vi "Get Control Absolute Position.vi"(8 "error in (no error)":errorcluster, 11 "Boolean in":refnum<vi>) -> (0 "error out":errorcluster, 2 "Absolute Position":T1)   [LabVIEW 2017, in "Hamburger Menu Library.lvlib"]
uses:
  Hamburger Menu Library.lvlib
  <vilib>/Utility/miscctls.llb/LVPositionTypeDef.ctl
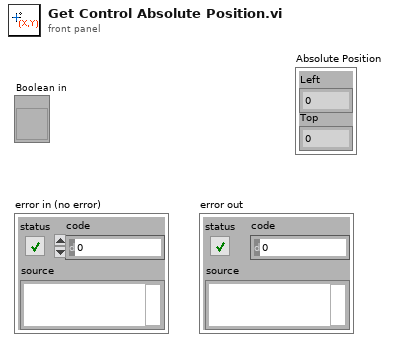
[diagram p1: front panel]
types:
  T1 = typedef "LVPositionTypeDef.ctl" = cluster{"Left":i32, "Top":i32}
  T2 = typedef "LVPointTypeDef.ctl" = cluster{"Horizontal":i16, "Vertical":i16}
  T3 = typedef "LVRectTypeDef.ctl" = cluster{"Left":i16, "Top":i16, "Right":i16, "Bottom":i16}
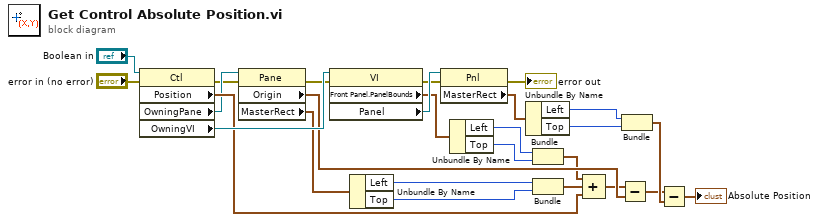
[diagram p0: block diagram]
diagram:
  n1 = property class="Ctl"(reference="Boolean in", error in="error in (no error)") -> (error out=w3:errorcluster, "Position"=w11:T1, "OwningPane"=w6:refnum<vi>, "OwningVI"=w22:refnum<vi>)  [unwired: 1 out]
  n2 = property class="Pane"(reference=w6, error in=w3) -> (error out=w2:errorcluster, "Origin"=w17:T2, "MasterRect"=w12:T3)  [unwired: 1 out]
  n3 = property class="VI"(reference=w22, error in=w2) -> (error out=w1:errorcluster, "Front Panel.PanelBounds"=w5:T3, "Panel"=w23:refnum<vi>)  [unwired: 1 out]
  n4 = Unbundle By Name(w12) -> ("Left"=w13:i16, "Top"=w14:i16)
  n5 = property class="Pnl"(reference=w23, error in=w1) -> (error out=→"error out":errorcluster, "MasterRect"=w21:T3)  [unwired: 1 out]
  n6 = Unbundle By Name(w5) -> ("Left"=w7:i16, "Top"=w8:i16)
  n7 = Unbundle By Name(w21) -> ("Left"=w20:i16, "Top"=w19:i16)
  n8 = Bundle("Left"=w7, "Top"=w8) -> (w9:cluster{"Left":i16, "Top":i16})  [unwired: 1 in]
  n9 = Bundle("Left"=w13, "Top"=w14) -> (w15:cluster{"Left":i16, "Top":i16})  [unwired: 1 in]
  n10 = Compound Arithmetic op=ADD(w9, w15, w11) -> (w16:T1)
  n11 = Subtract(x=w16, y=w17) -> (x-y=w18:T1)
  n12 = Bundle("Left"=w20, "Top"=w19) -> (w24:cluster{"Left":i16, "Top":i16})  [unwired: 1 in]
  n13 = Subtract(x=w18, y=w24) -> (x-y=→"Absolute Position":T1)
